vi "Create Test Executive.vi"(8 "error in (no error)":errorcluster, 10 "Create Test Executive":T1, 11 "Test Executive Builder Model in":refnum<class "Test Executive Builder Model.lvclass">) -> (0 "error out":errorcluster, 3 "Test Executive Builder Model out":refnum<class "Test Executive Builder Model.lvclass">, 5 "Unique ID":string)   [LabVIEW 2019, in "Test Executive Builder Model.lvclass"]
uses:
  <vilib>/gpm_packages/@cs/Test-executive-builder/Source/Test Executive Builder Model/Test Executive Builder Model/Test Executive Builder Model.lvclass
  C:/Program Files/National Instruments/LabVIEW 2019/vi.lib/ActorFramework/Actor/Actor.lvclass
  <vilib>/gpm_packages/@cs/Test-executive-builder/Source/Application Dependencies/Create Test Executive.ctl
  <vilib>/gpm_packages/@cs/Test-executive-builder/Source/Test Executive Builder Model/Test Executive Builder Model/Test Executive Builder Model.lvclass/Test Executive Builder Model.ctl
  <vilib>/ActorFramework/Actor/Actor.lvclass/Actor.ctl
  <vilib>/ActorFramework/Message Enqueuer/Message Enqueuer.lvclass/Message Enqueuer.ctl
  <vilib>/gpm_packages/@cs/Test-executive-builder/Source/Test Executive Builder Model/Test Executive Builder Model Messages/Evaluate Save Test Executive Msg/Evaluate Save Test Executive Msg.lvclass/Evaluate Save Test Executive Msg.ctl
  <vilib>/ActorFramework/Message Enqueuer/Init from Existing Queue.vi
  <vilib>/ActorFramework/Message Enqueuer/Enqueue.vi
  <vilib>/gpm_packages/@cs/Test-executive-builder/Source/Test Executive Builder Model/Test Executive Builder Model Messages/Evaluate Save Test Executive Msg/Evaluate Save Test Executive Msg.lvclass
  C:/Program Files/National Instruments/LabVIEW 2019/vi.lib/ActorFramework/Message/Message.lvclass
  <vilib>/gpm_packages/@cs/Test-executive-builder/Source/Test Executive Builder Model/Test Executive Builder Model Messages/Redraw Tree Msg/Redraw Tree Msg.lvclass
  <vilib>/ActorFramework/Message Priority Queue/Priority Enqueue.vi
  <vilib>/ActorFramework/Message Enqueuer/Message Enqueuer.lvclass
  <vilib>/gpm_packages/@cs/test-executive/Source/Test Executive/TestExecutive Ref/TestExecutive Ref.lvclass
  <vilib>/ActorFramework/Actor/Actor.lvclass
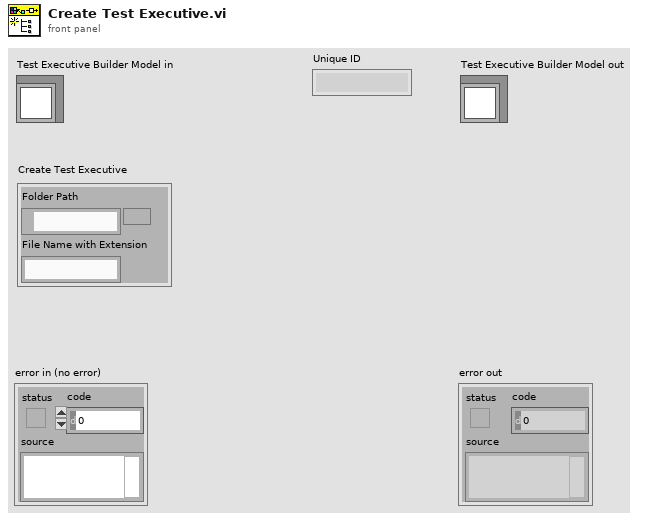
[diagram p1: front panel]
types:
  T1 = typedef "Create Test Executive.ctl" = cluster{"Folder Path":path, "File Name with Extension":string}
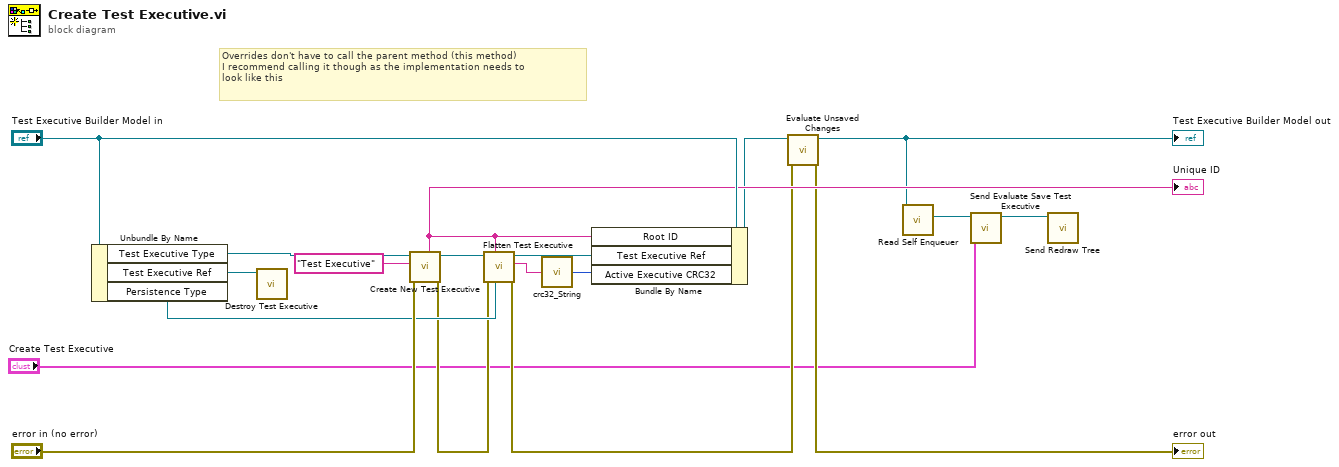
[diagram p0: block diagram]
diagram:
  # "Overrides don't have to call the parent method (this method)\nI recommend calling it though as the implementation needs to\nlook like this"
  n1 = Unbundle By Name("Test Executive Builder Model in") -> ("Test Executive Type"=w18:refnum<class "ITest Executive.lvclass">, "Test Executive Ref"=w19:refnum<data-value>, "Persistence Type"=w10:refnum<class "IPersist.lvclass">)
  n2 = call <vilib>:"Destroy Test Executive.vi"("Test Executive Ref"=w19) -> ()  [unwired: 10 in, 1 out]
  n3 = call <vilib>:"Create New Test Executive.vi"("error in (no error)"="error in (no error)", "Name"="Test Executive", "Test Executive"=w18) -> ("error out"=w9:errorcluster, "Test Executive Ref"=w13:refnum<data-value>, "Test Executive ID out"=w11:string)  [unwired: 6 in]
  "Unique ID" <- w11
  n4 = call <vilib>:"Flatten Test Executive.vi"("Persistence in"=w10, "Root ID"=w11, "error in (no error)"=w9, "Test Executive Ref"=w13) -> ("error out"=w6:errorcluster, "Flattened Test Executive"=w14:string, "Test Executive Ref out"=w12:refnum<data-value>)  [unwired: 5 in]
  n5 = call <vilib>:"crc32_String.vi"("String in"=w14) -> ("CRC32"=w8:u32)  [unwired: 1 in]
  n6 = Bundle By Name(cluster="Test Executive Builder Model in", "Root ID"=w11, "Test Executive Ref"=w12, "Active Executive CRC32"=w8) -> (w7:refnum<class "Test Executive Builder Model.lvclass">)
  n7 = call-dynamic "Evaluate Unsaved Changes.vi"("error in (no error)"=w6, "Test Executive Builder Model in"=w7) -> ("error out"=→"error out":errorcluster, "Test Executive Builder Model out"=w5:refnum<class "Test Executive Builder Model.lvclass">)  [unwired: 8 in]
  "Test Executive Builder Model out" <- w5
  n8 = call <vilib>:"Read Self Enqueuer.vi"("Actor"=w5) -> ("Self Enqueuer"=w3:refnum<class "Message Enqueuer.lvclass">)  [unwired: 10 in]
  n9 = call <vilib>:"Send Evaluate Save Test Executive.vi"("Create Test Executive"="Create Test Executive", "Message Enqueuer"=w3) -> ("Message Enqueuer out"=w2:refnum<class "Message Enqueuer.lvclass">)  [unwired: 8 in, 1 out]
  n10 = call <vilib>:"Send Redraw Tree.vi"("Message Enqueuer"=w2) -> ()  [unwired: 9 in, 2 out]
